vi "ingest.tabular_add_file_tag.vi"(8 "error in":errorcluster, 9 "value":string, 10 "tag":string, 11 "TabularIngestStaging in":refnum<class "TabularIngestStaging.lvclass">) -> (0 "error out":errorcluster, 3 "TabularIngestStaging out":refnum<class "TabularIngestStaging.lvclass">)   [LabVIEW 2020, in "TabularIngestStaging.lvclass"]
doc: "Applies a fixed tag and value to every row ingested from the file."
uses:
  TabularIngestStaging.lvclass
  TabularIngestStaging.lvclass/TabularIngestStaging.ctl
  client.lvlib
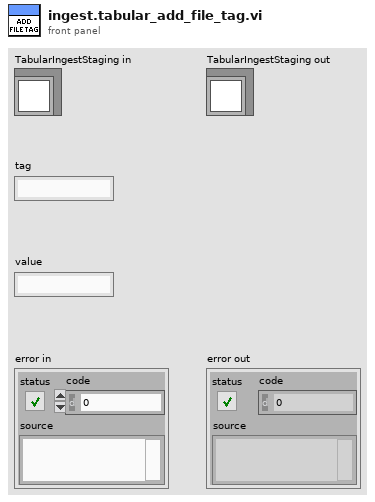
[diagram p1: front panel]
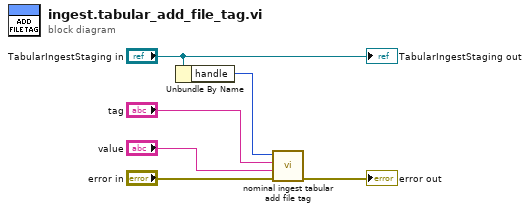
[diagram p0: block diagram]
diagram:
  n1 = Unbundle By Name("TabularIngestStaging in") -> ("handle"=w4:i32)
  n2 = call "nominal ingest tabular add file tag.vi"("error in (no error)"="error in", "value"="value", "tag"="tag", "staging"=w4) -> ("error out"=→"error out":errorcluster)  [unwired: 6 in, 1 out]
  "TabularIngestStaging out" <- "TabularIngestStaging in"
